vi "GEA2_ICP_Washer_SM.vi"(0 "ComPort":refnum<visa-resource-name>="COM1", 1 "Destination Address":u8=37 format="%.0x", 2 "Source Address":u8=229 format="%.0x", 3 "Mode":T2, 5 "Filter on Destination":bool, 7 "Read Bus Idle Timeout":u32=42, 9 "Byte Data":u8[](array[numeric]) format="%02x", 11 "Error In":errorcluster, 12 "Partial Message Start":u8[](array[numeric]) format="%02x", 13 "Command":u8(ring)=2 items=["CMD_Entry_Command", "CMD_Load_Control", "RQST_Input_Status", "CMD_LED_Control", "RQST_Encoder_Position_Status", "RQST_A2D_Status", "RQST_Switch_States_Status", "CMD_Buzzer_Control", "CMD_Shift_to_Spin", "CMD_Shift_to_Agitate", "RQST_Mode_Shift_Complete_Status", "CMD_Control_Inverter", "CMD_Spin_Action", "CMD_Agitate_Action", "RQST_Total_Switch_Status", "RQST_Total_Encoder_Status", "CMD_Test_Eeprom", "RQST_Eeprom_Test_Status", "CMD_Power_Mode", "RQST_Error_Status", "RQST_Get_Version", "CMD_Set_Personality", "RQST_Get_Personality", "CMD_Serial_Number", "RQST_Serial_Number_Status", "CMD_Model_Number", "RQST_Model_Number_Status", "CMD_Enter_Boot_Loader", "CMD_Enable_Debug_Log"]) -> (4 "Good Responses":cluster{"Bytes Data":u8[]}[](array[cluster]) {"Bytes Data" format="%02x"}, 10 "WriteOK":bool, 14 "Partial Message Out":u8[](array[numeric]) format="%.0x", 15 "Error Out":errorcluster)   [LabVIEW 2011]
uses:
  GEA2 Washer Interface Ctrl.ctl
  Dryer Wilt/Dryer Commands.ctl
  Hybrid Water Heater/HEWH Error Enumeration.ctl
  <vilib>/Instr/_visa.llb/VISA Configure Serial Port (Instr).vi
panel:
  in  "Read Continuous":bool
  out "CRC Match":bool
  in  "Tab Control":T1(tab)
  in  "Send Command":bool
  out "Command Bytes":u8[](array[numeric])=[226, 96, 8, 128, 86, 123, 137, 227] format="%.0x"
  out "Info":string
  in  "Read?":bool
  out "Length":u8
  out "Source Read":u8 format="%.0x"
  out "Destination Read":u8 format="%.0x"
  out "DataReturned":u8[](array[numeric]) format="%.0x"
  out "ReadArray":u8[](array[numeric]) format="%.0x"
  out "Bytes At Port":u32=40
  out "CRCRead":u8[](array[numeric]) format="%.0x"
  out "CRC Calc":u8[](array[numeric]) format="%.0x"
  out "Timeout":bool
  out "Num Messages":dbl
  out "Read Message Count":dbl
  out "CRCArray":u8[](array[numeric]) format="%.0x"
  out "Time Array":i32[](array[numeric])
  out "Tdiff":i32[](array[numeric])
  out "tStart":u32
  out "State Array":string[](array[string])
  out "Total mS":i32
  in  "Debug":bool
  out "Read_ACK":bool
  out "Message for Me":bool
  out "Partial Message":bool
  out "Current Start of Message Index":i32
  in  "Exit":bool
  # "Use only in Send Byte\nData Mode"
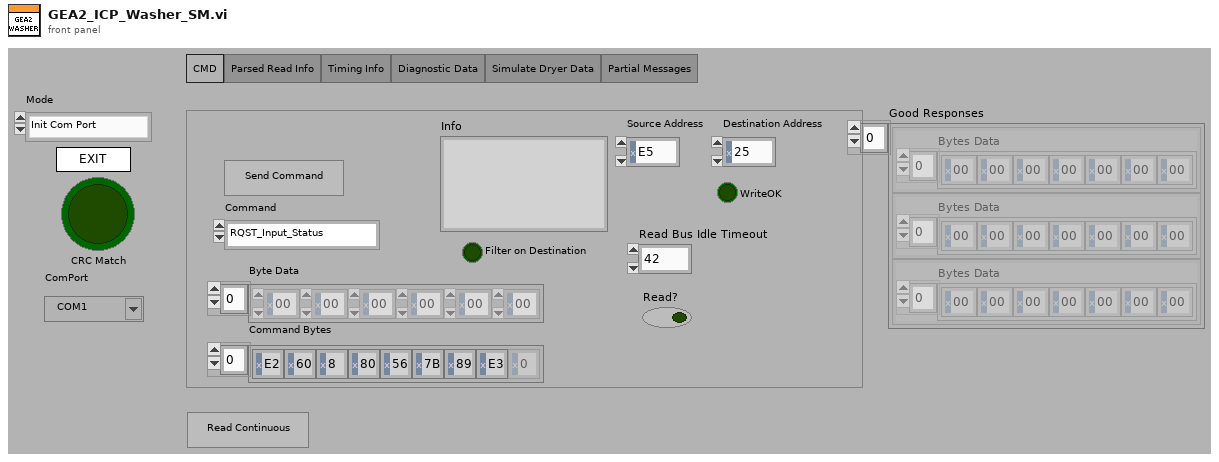
[diagram p1: front panel]
types:
  T1 = enum32{"CMD", "Parsed Read Info", "Timing Info", "Diagnostic Data", "Simulate Dryer Data", "Partial Messages"}
  T2 = typedef "GEA2 Washer Interface Ctrl.ctl" = enum16{"Init Com Port", "SendCMD", "ReadPort", "Close Port", "Send Byte Data", "Read Continuous"}
  T3 = enum32{"invalid app kind", "Development System", "Run Time System", "Student Edition", "Embedded LabVIEW", "Evaluation", "Custom"}
  T4 = enum32{"Invalid", "Standard", "Closed", "Hidden", "Minimized", "Maximized"}
  T5 = typedef "HEWH Error Enumeration.ctl" = enum16{"No Error", "GEA2 Send ACK Mismatch", "GEA2 STX", "GEA2 ETX", "GEA2 CRC Mismatch", "GEA2 ReadACK", "RTD In Range Error", "Fail Mean Tank Temp", "No Flow Config Data Found", "Failed Flow During Purge", "Temp During Purge", "Confirm IF Stop Fail", "Init Draw: TC_1 Out of Range", "Flow = 0 During Draw after 20s"}
  T6 = typedef "Dryer Commands.ctl" = u8
  T7 = cluster{"Core":cluster{"Current VI Reference":refnum<vi>, "Close Panel on Exit?":bool}, "ComPort":refnum<visa-resource-name>, "ReadArray":u8[], "Partial Message Start":u8[], "CRCArray":u8[], "Bytes Remaining":u8, "CRCRead":u8[], "CRC":bool, "Dryer Command":T6, "Error Out Flag":bool, "Bytes Data":u8[], "Current Read Index":i32, "Total Bytes Read":i32, "Reset MSG Count":bool, "ACK":bool, "ReadCM1Flag":bool, "ReadCM2Flag":bool, "Reset Pulse":bool, "Good Responses":cluster{"Bytes Data":u8[]}[]}
  T8 = cluster{"Current VI Reference":refnum<vi>, "Close Panel on Exit?":bool}
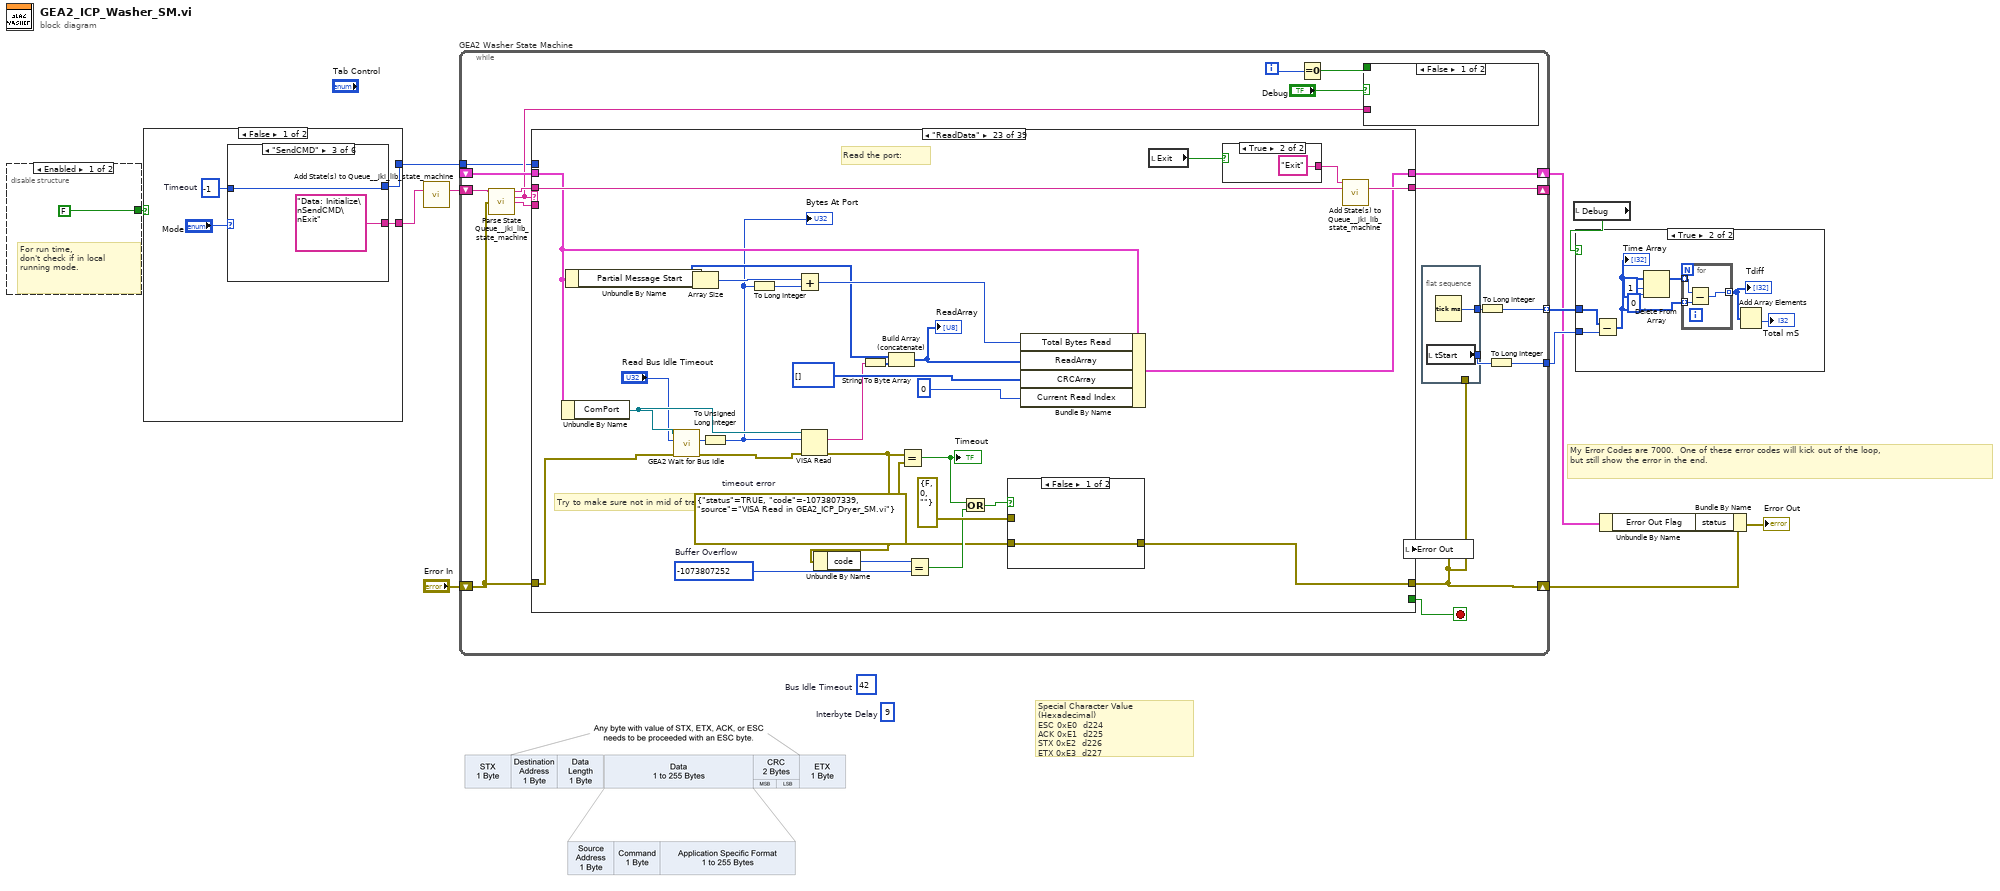
[diagram p0: block diagram]
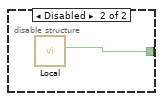
[diagram p2: hidden frame]
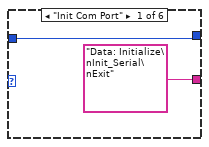
[diagram p3: hidden frame]
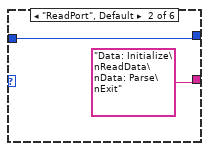
[diagram p4: hidden frame]
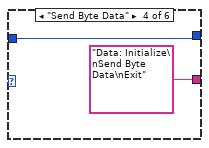
[diagram p5: hidden frame]
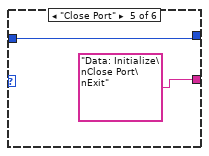
[diagram p6: hidden frame]
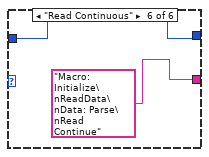
[diagram p7: hidden frame]
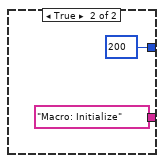
[diagram p8: hidden frame]
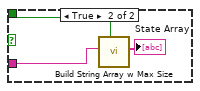
[diagram p10: hidden frame]
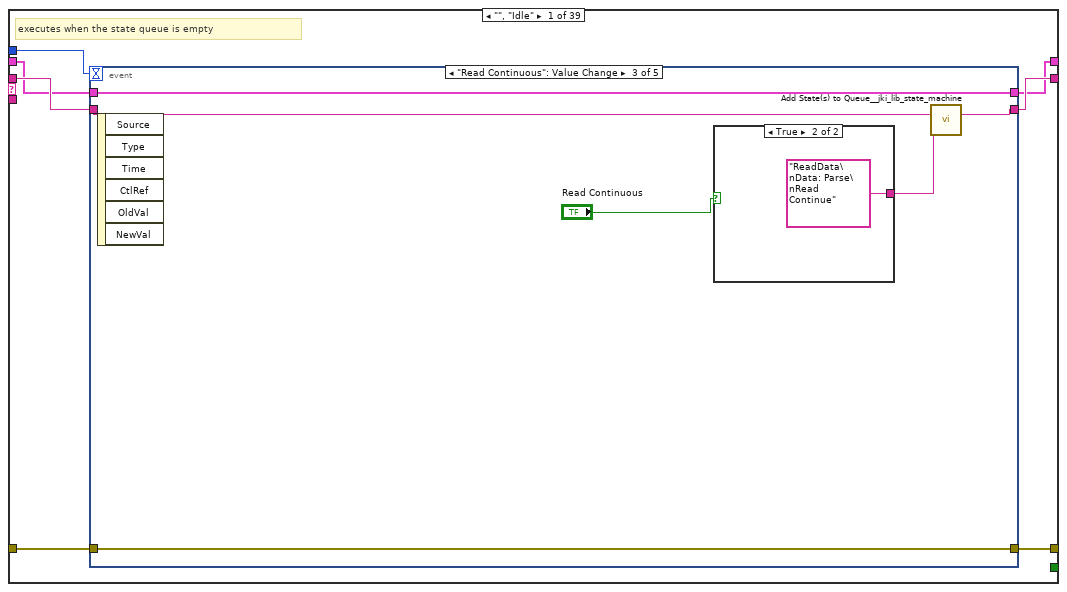
[diagram p11: hidden frame]
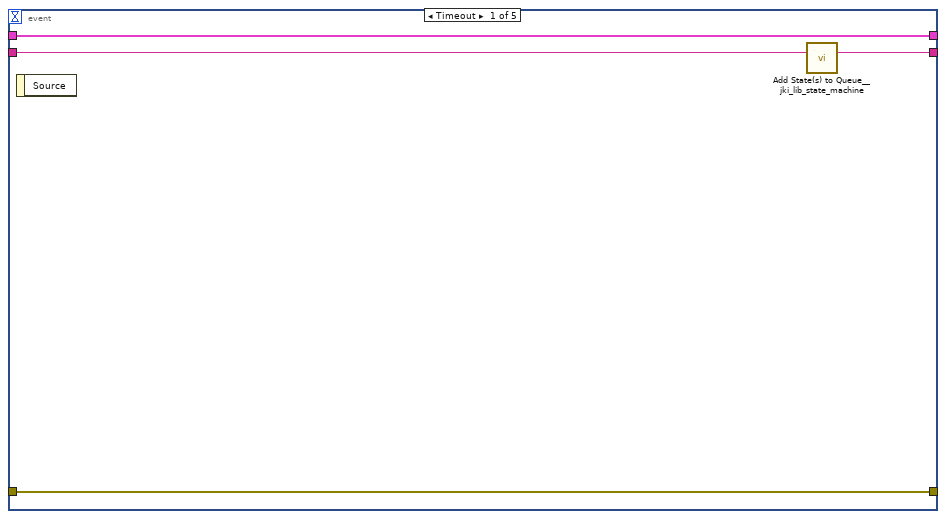
[diagram p12: hidden frame]
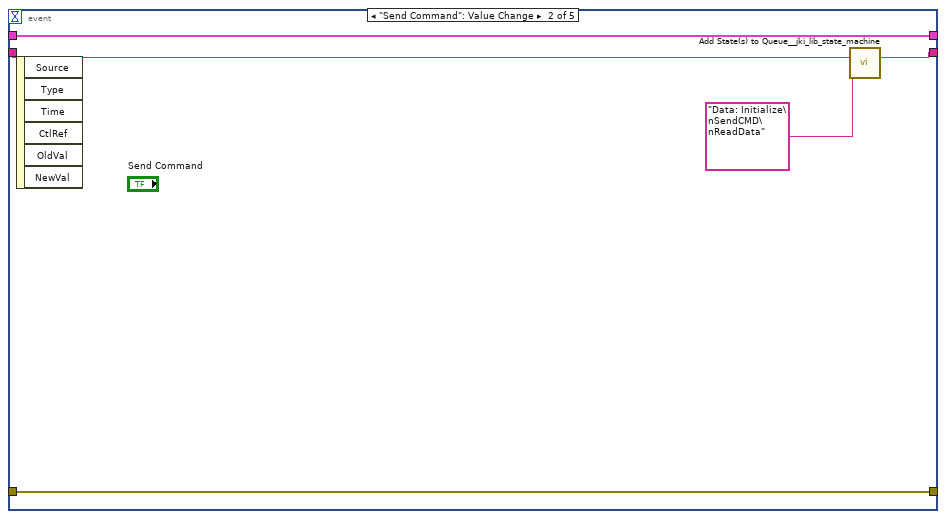
[diagram p13: hidden frame]
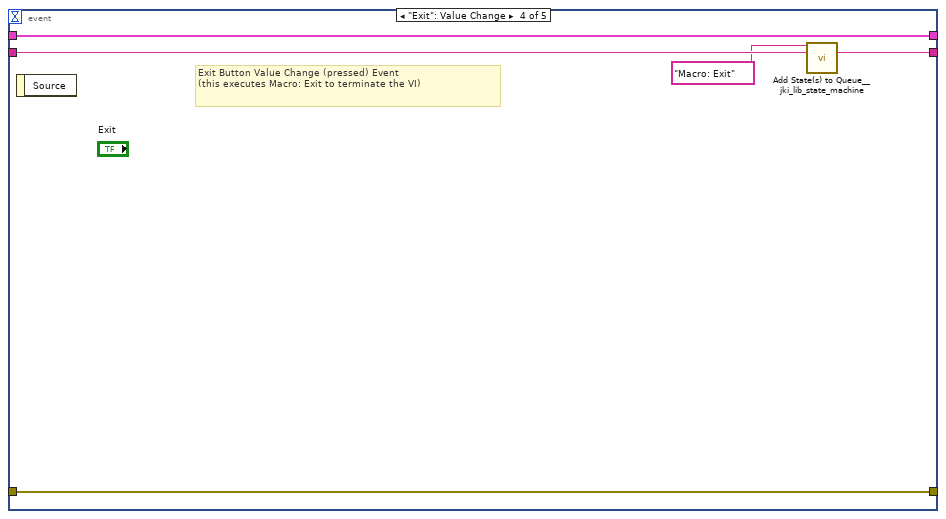
[diagram p15: hidden frame]
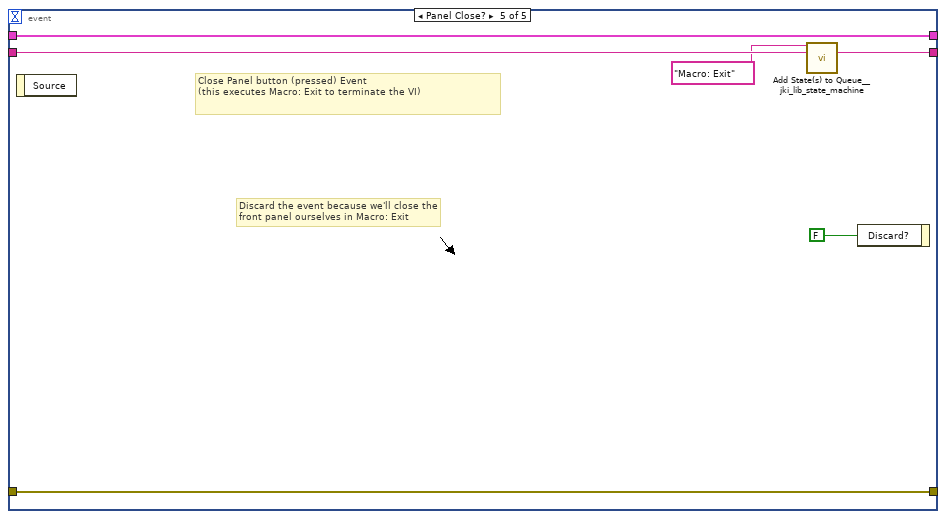
[diagram p16: hidden frame]
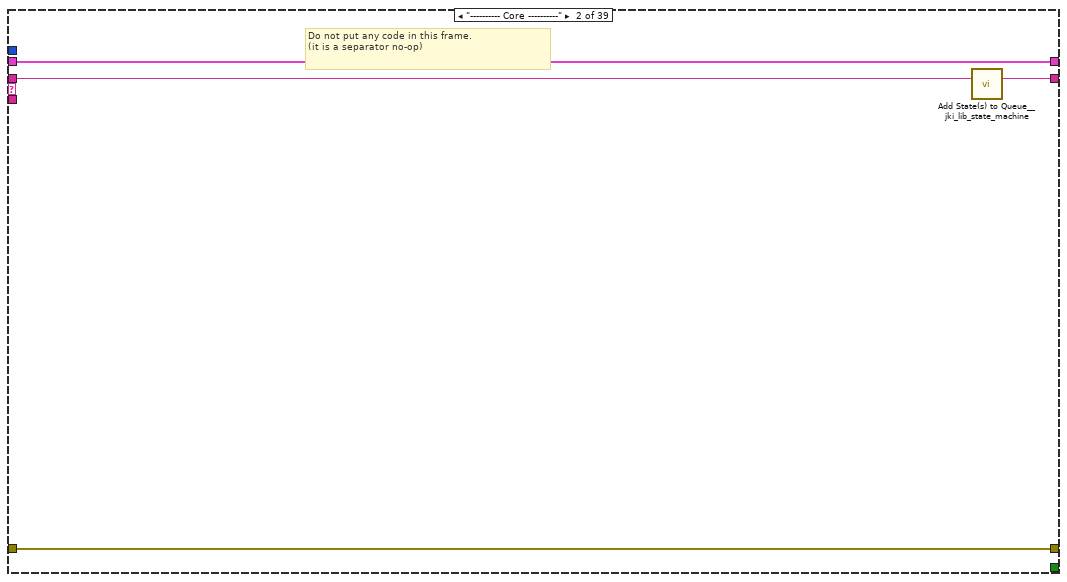
[diagram p17: hidden frame]
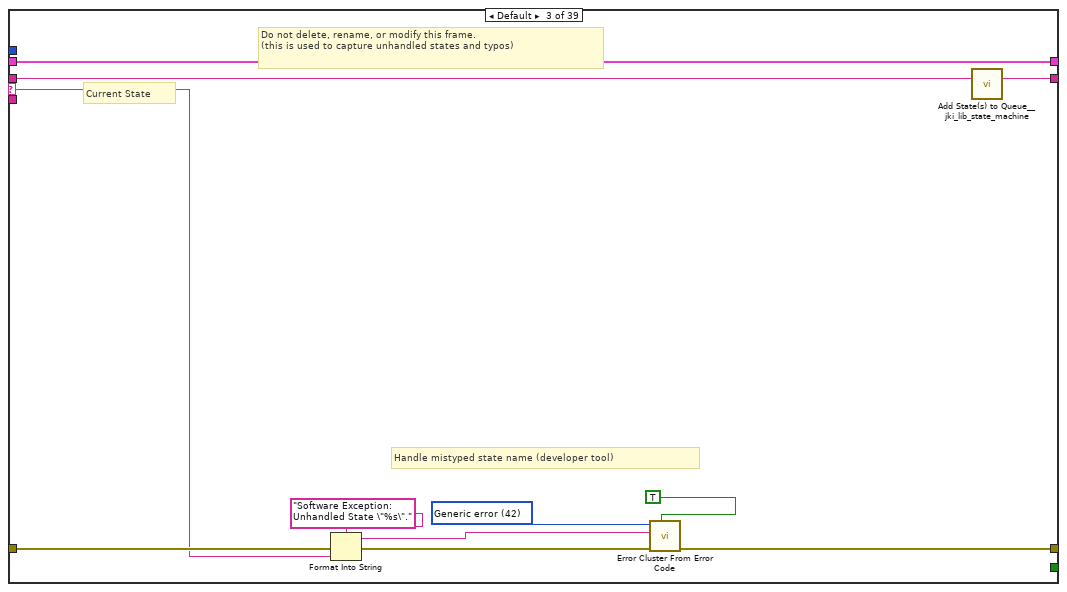
[diagram p18: hidden frame]
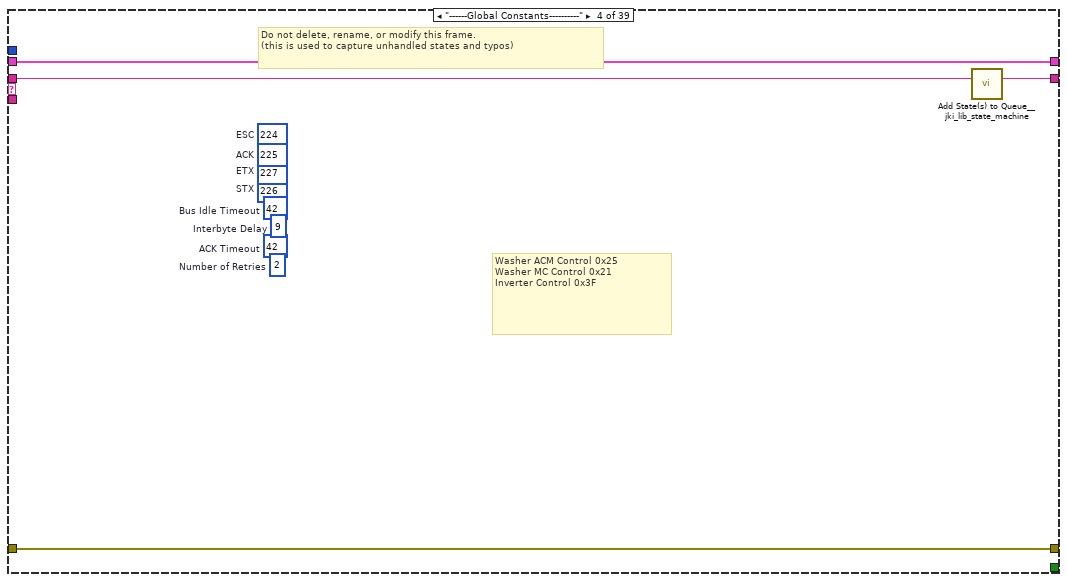
[diagram p19: hidden frame]
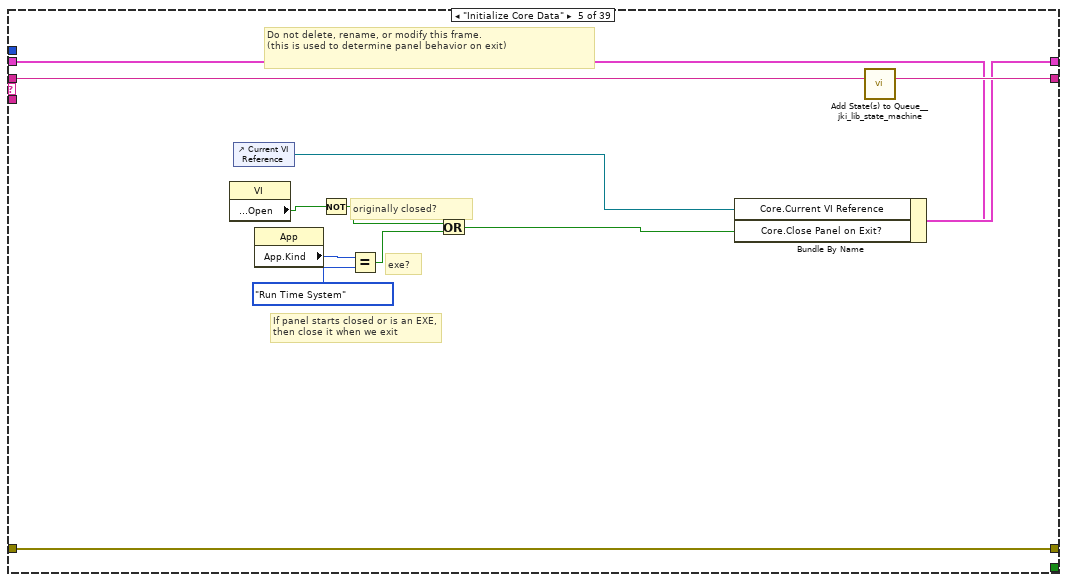
[diagram p20: hidden frame]
diagram:
  (unwired) 9  # Interbyte Delay
  (unwired) 42  # Bus Idle Timeout
  # "Special Character\tValue (Hexadecimal)\nESC\t0xE0  d224\nACK\t0xE1  d225\nSTX\t0xE2  d226\nETX\t0xE3  d227"
  # "My Error Codes are 7000.  One of these error codes will kick out of the loop,\nbut still show the error in the end."
  n1 = disable-structure shown="Enabled" {
    disable-tunnel: [FALSE w14] -> w1
    frame Enabled {
      # "For run time,\ndon't check if in local\nrunning mode."
    }
    frame Disabled {
      n2 = call "Local.vi"() -> ("Local?"=w14:bool)  [unwired: 11 in]
    }
  }
  n3 = case shown="False" w1 {
    tunnel: [w17 200 ("Timeout")] -> w4
    tunnel: [w15 "Macro: Initialize"] -> w2
    frame False {
      w16 = -1  # Timeout
      n4 = case shown="\"SendCMD\"" "Mode" {
        tunnel: ["Data: Initialize\nInit_Serial\nExit" "Data: Initialize\nReadData\nData: Parse\nExit" "Data: Initialize\nSendCMD\nExit" "Data: Initialize\nSend Byte Data\nExit" "Data: Initialize\nClose Port\nExit" "Macro: Initialize\nReadData\nData: Parse\nRead Continue"] -> w15
        tunnel: [w19 w21 w23 w25 w27 w30] -> w17
        tunnel: w16 -> [w19 w21 w23 w25 w27 w30]
        frame "Init Com Port" {
        }
        frame "ReadPort", Default {
        }
        frame "SendCMD" {
        }
        frame "Send Byte Data" {
        }
        frame "Close Port" {
        }
        frame "Read Continuous" {
        }
      }
    }
    frame True {
    }
  }
  n5 = call <vilib>:"Add State(s) to Queue__jki_lib_state_machine.vi"("State(s) in (\"\")"=w2) -> ("States Out"=w12:string)  [unwired: 14 in]
  n6 = while "GEA2 Washer State Machine" {
    shift-right: [w46] -> w6
    shift-left: _ -> [w45]
    shift-right: [w42] -> w10
    shift-left: "Error In" -> [w44]
    shift-right: [w43] -> _
    shift-left: w12 -> [w48]
    tunnel: [w39] -> w9 mode=indexing
    tunnel: [w38] -> w8
    tunnel: w4 -> [w36]
    i -> [w34]
    stop <- w47 stop-if-true
    n7 = call <vilib>:"Parse State Queue__jki_lib_state_machine.vi"("State Queue"=w48, "Error In (no error)"=w44) -> ("Remaining States"=w50:string, "Current State"=w37:string, "Arguments"=w49:string)  [unwired: 11 in]
    n8 = case shown="\"ReadData\"" w37 {
      selector: w37 -> [_ _ w94 _ _ _ _ _ _ _ _ _ _ _ _ _ _ _ _ _ _ _ _ _ _ _ _ _ _ _ _ _ _ _ _ _ _ _ _]
      tunnel: w50 -> [w62 w93 w98 w108 w120 w136 w138 w149 w178 w185 w190 w194 w200 w211 w237 w243 w248 w259 w276 w297 w346 w383 w415 w422 w431 w452 w484 w503 w547 w576 w597 w618 w634 w647 w660 w691 w713 w727 w734]
      tunnel: w49 -> [_ _ _ _ _ _ _ _ _ _ _ _ w195 w205 _ _ _ _ _ _ _ _ _ _ _ _ _ _ _ _ _ _ _ _ _ _ _ _ _]
      tunnel: w45 -> [w60 w90 w96 w106 w111 w132 w141 w146 _ w182 w187 w192 w198 w207 w234 w240 w245 w256 w273 w294 w323 w365 w397 w419 w425 w450 w482 w519 w545 w574 w595 w616 w629 w645 w655 w683 w702 w721 w732]
      tunnel: [w59 w91 w100 w105 w117 w134 w142 w147 w164 w180 w188 w191 w196 w208 w235 w241 w246 w257 w274 w295 w309 w355 w400 w420 w429 w447 w478 w516 w539 w570 w591 w612 w627 w642 w656 w689 w711 w725 w733] -> w42
      tunnel: w44 -> [w58 w91 w99 w105 w117 w128 w142 w147 w164 w183 w188 w191 w197 w209 w235 w241 w246 w257 w263 w290 w327 w369 w391 w420 w429 w445 w478 w516 w539 w570 w591 w612 w632 w639 w658 w689 w711 w725 w733]
      tunnel: [w61 w92 w97 w107 w119 w135 w143 w148 w177 w184 w189 w193 w199 w210 w236 w242 w247 w258 w275 w296 w345 w382 w414 w421 w430 w451 w483 w520 w546 w575 w596 w617 w633 w646 w659 w690 w712 w726 w735] -> w43
      tunnel: [_ _ _ _ _ _ w139 _ _ _ _ _ _ _ _ _ _ _ _ _ _ _ _ _ _ _ _ _ _ _ _ _ _ _ _ _ _ _ _] -> w47
      tunnel: [w57 w90 w96 w106 w118 w131 w141 w146 w176 w182 w187 w192 w198 w207 w234 w240 w245 w256 w272 w293 w323 w365 w407 w419 w424 w449 w481 w518 w544 w573 w594 w615 w628 w644 w655 w682 w701 w724 w732] -> w46
      tunnel: w36 -> [w56 _ _ _ _ _ _ _ _ _ _ _ _ _ _ _ _ _ _ _ _ _ _ _ _ _ _ _ _ _ _ _ _ _ _ _ _ _ _]
      frame "", "Idle" {
        # "executes when the state queue is empty"
        n9 = event shown="[2] \"Read Continuous\": Value Change" {
          selector: _ -> [_ _ _ _ _]
          dyn-events: _ -> [_ _ _ _ _]
          timeout: w56 -> [_ _ _ _ _]
          tunnel: w62 -> [w66 w69 w75 w83 w89]
          tunnel: [w65 w70 w76 w82 w88] -> w61
          tunnel: w60 -> [w63 w71 w77 w80 w86]
          tunnel: [w64 w67 w73 w81 w87] -> w59
          tunnel: w58 -> [w64 w67 w73 w81 w87]
          tunnel: [w63 w71 w77 w80 w86] -> w57
          event Timeout {
            n10 = event-data() -> ()  [unwired: 1 in, 1 out]
            n11 = call <vilib>:"Add State(s) to Queue__jki_lib_state_machine.vi"("State(s) in (\"\")"=w66) -> ("States Out"=w65:string)  [unwired: 14 in]
          }
          event "Send Command": Value Change {
            n12 = event-data() -> ()  [unwired: 1 in, 6 out]
            n13 = call <vilib>:"Add State(s) to Queue__jki_lib_state_machine.vi"("State(s) in (\"\")"=w69, "State(s) at Back (\"\")"="Data: Initialize\nSendCMD\nReadData") -> ("States Out"=w70:string)  [unwired: 13 in]
          }
          event "Read Continuous": Value Change {
            n14 = event-data() -> ()  [unwired: 1 in, 6 out]
            n15 = case shown="True" "Read Continuous" {
              tunnel: [_ "ReadData\nData: Parse\nRead Continue"] -> w74
              frame False {
              }
              frame True {
              }
            }
            n16 = call <vilib>:"Add State(s) to Queue__jki_lib_state_machine.vi"("State(s) in (\"\")"=w75, "State(s) at Back (\"\")"=w74) -> ("States Out"=w76:string)  [unwired: 13 in]
          }
          event "Exit": Value Change {
            # "Exit Button Value Change (pressed) Event\n(this executes Macro: Exit to terminate the VI)"
            n17 = event-data() -> ()  [unwired: 1 in, 1 out]
            n18 = call <vilib>:"Add State(s) to Queue__jki_lib_state_machine.vi"("State(s) in Front (\"\")"="Macro: Exit", "State(s) in (\"\")"=w83) -> ("States Out"=w82:string)  [unwired: 13 in]
          }
          event Panel Close? {
            # "Discard the event because we'll close the front panel ourselves in Macro: Exit"
            # "Close Panel button (pressed) Event\n(this executes Macro: Exit to terminate the VI)"
            n19 = event-data() -> ()  [unwired: 1 in, 1 out]
            n20 = call <vilib>:"Add State(s) to Queue__jki_lib_state_machine.vi"("State(s) in Front (\"\")"="Macro: Exit", "State(s) in (\"\")"=w89) -> ("States Out"=w88:string)  [unwired: 13 in]
            n21 = event-data("Discard?"=FALSE) -> ()  [unwired: 1 in, 1 out]
          }
        }
      }
      frame "---------- Core ----------" {
        # "Do not put any code in this frame.\n(it is a separator no-op)"
        n22 = call <vilib>:"Add State(s) to Queue__jki_lib_state_machine.vi"("State(s) in (\"\")"=w93) -> ("States Out"=w92:string)  [unwired: 14 in]
      }
      frame Default {
        w103 = 42 items=["No error", "Argument error", "Memory is full", "Out of zone", "End of file", "File already open", "Generic file I/O error", "File not found", "File permission error", "Disk is full", "Duplicate path", "Too many files open", "System feature not enabled", "Resource file not found", "Cannot add resource", "Resource not found", "Image not found", "Image memory error", "Pen does not exist", "Config type invalid", "Config token not found", "Config parse error", "Config memory error", "Bad external code format", "Bad external code offset", "External code not present", "Null window", "Destroy window error", "Null menu", "Print aborted", "Bad print record", "Print driver error", "Windows error during printing", "Memory error during printing", "Print dialog error", "Generic print error", "Invalid device refnum", "Device not found", "Device parameter error", "Device unit error", "Cannot open device", "Device call aborted", "Generic error", "Cancelled by user", "Object ID too low", "Object ID too high", "Object not in heap", "Unknown heap", "Unknown object (invalid DefProc)", "Unknown object (DefProc not in table)", "Message out of range", "Invalid (null) method", "Unknown message", "Manager call not supported", "Bad address", "Network operation in progress", "Network operation timed out", "Connection is busy", "Network attribute not supported", "Network error", "Address in use", "System out of memory", "Connection aborted", "Connection refused", "Not connected", "Already connected", "Connection closed", "Initialization error (interapplication manager)", "Bad occurrence", "Wait on unbound occurrence handler", "Occurrence queue overflow", "Datalog type conflict", "Unused", "Unrecognized type (interapplication manager)", "Memory corrupt", "Failed to make temporary DLL", "Old CIN version", "Drag socket not found", "Failed to load drop-object", "Failed to register OLE object", "Failed to release OLE object", "Format specifier type mismatch", "Unknown format specifier", "Too few format specifiers", "Too many format specifiers", "Scan failed", "Newer CIN version", "Error converting to variant", "Runtime menu error", "Password tampered", "Variant attribute not found", "Incompatible variant data type", "Event data is not available", "Event Store is not present", "Occurrence is not found", "Event Queue is not created", "Event info is not available", "Refnum passed is NULL", "Error retrieving Class GUID", "Error retrieving CoClass GUID", "Error retrieving TypeLib GUID.", "Bad built application magic bytes.", "Specific driver is different from the specific driver associated with the Logical Name.", "There is no session opened to the class driver.", "Max Error", "MAX - Error with config objects", "MAX - Error loading configuration", "MAX - Group not supported"]
        # "Current State"
        # "Do not delete, rename, or modify this frame.\n(this is used to capture unhandled states and typos)"
        # "Handle mistyped state name (developer tool)"
        n23 = Format Into String(format string="Software Exception: Unhandled State \"%s\"." ("message"), error in=w99, w94) -> (resulting string=w102:string, error out=w101:errorcluster)  [unwired: 1 in]
        n24 = call <vilib>:"Error Cluster From Error Code.vi"("show call chain? (False)"=TRUE, "error in (no error)"=w101, "error message (\"\")"=w102, "error code (0)"=w103) -> ("error out"=w100:errorcluster)  [unwired: 5 in]
        n25 = call <vilib>:"Add State(s) to Queue__jki_lib_state_machine.vi"("State(s) in (\"\")"=w98) -> ("States Out"=w97:string)  [unwired: 14 in]
      }
      frame "------Global Constants----------" {
        (unwired) u8 224  # ESC
        (unwired) 2  # Number of Retries
        (unwired) 42  # ACK Timeout
        (unwired) 9  # Interbyte Delay
        (unwired) 42  # Bus Idle Timeout
        (unwired) u8 226  # STX
        (unwired) u8 227  # ETX
        (unwired) u8 225  # ACK
        # "Washer ACM Control\t0x25\nWasher MC Control\t0x21\nInverter Control\t0x3F"
        # "Do not delete, rename, or modify this frame.\n(this is used to capture unhandled states and typos)"
        n26 = call <vilib>:"Add State(s) to Queue__jki_lib_state_machine.vi"("State(s) in (\"\")"=w108) -> ("States Out"=w107:string)  [unwired: 14 in]
      }
      frame "Initialize Core Data" {
        # "Do not delete, rename, or modify this frame.\n(this is used to determine panel behavior on exit)"
        # "originally closed?"
        # "exe?"
        # "If panel starts closed or is an EXE, then close it when we exit"
        n27 = property class="VI"() -> ("Front Panel.Open"=w116:bool)  [unwired: 2 in, 2 out]
        n28 = control-ref of="Current VI Reference"() -> (w109:refnum<vi>)
        n29 = property class="App"() -> ("App.Kind"=w115:T3)  [unwired: 2 in, 2 out]
        n30 = Not(x=w116) -> (.not. x?=w113:bool)
        n31 = Equal?(x=w115, y=T3."Run Time System" ("Application:Kind")) -> (x = y?=w112:bool)
        n32 = Or(x=w113, y=w112) -> (x .or. y?=w110:bool)
        n33 = Bundle By Name(cluster=w111, "Core.Current VI Reference"=w109, "Core.Close Panel on Exit?"=w110) -> (w118:T7)
        n34 = call <vilib>:"Add State(s) to Queue__jki_lib_state_machine.vi"("State(s) in (\"\")"=w120) -> ("States Out"=w119:string)  [unwired: 14 in]
      }
      frame "Error Handler" {
        # "State Machine Does not handle having an error status = true."
        n35 = local read "ReadArray"() -> (w125:u8[])
        n36 = Unbundle By Name(w128) -> ("source"=w127:string)
        n37 = Number To Hexadecimal String(2:w125) -> (0:w124:string[])  [unwired: 1 in]
        n38 = Array To Spreadsheet String(array=w124, 3:"" ("format string")) -> (spreadsheet string=w122:string)  [unwired: 1 in]
        n39 = Concatenate Strings(w127, ":: BYTES :: " ("string"), w122) -> (w121:string)
        n40 = Bundle By Name(cluster=w132, "Error Out Flag"=TRUE) -> (w131:T7)
        n41 = Bundle By Name(cluster=w128, "source"=w121, "status"=FALSE) -> (w134:errorcluster)
        n42 = call <vilib>:"Add State(s) to Queue__jki_lib_state_machine.vi"("State(s) in Front (\"\")"="Exit", "State(s) in (\"\")"=w136) -> ("States Out"=w135:string)  [unwired: 13 in]
      }
      frame "Exit" {
        # "Do not put any code in this frame.\n(No errors that occur here will be handled.)"
        n43 = local read "Mode"() -> (w140:T2)
        n44 = case shown="\"Init Com Port\", Default" w140 {
          tunnel: [TRUE] -> w139
          tunnel: w138 -> [w144]
          tunnel: [w144] -> w137
          frame "Init Com Port", Default {
          }
        }
        n45 = call <vilib>:"Add State(s) to Queue__jki_lib_state_machine.vi"("State(s) in (\"\")"=w137) -> ("States Out"=w143:string)  [unwired: 14 in]
      }
      frame "---------- Data ----------" {
        # "Do not put any code in this frame.\n(It is a separator no-op. You can make a copy of this frame to create a new Data frame)"
        n46 = call <vilib>:"Add State(s) to Queue__jki_lib_state_machine.vi"("State(s) in (\"\")"=w149) -> ("States Out"=w148:string)  [unwired: 14 in]
      }
      frame "Data: Initialize" {
        w150 = cluster{"Bytes Data":u8[]}[] []  # Good Responses
        w151 = FALSE ("Start Pressed")
        w154 = TRUE  # Reset Pulse
        w156 = FALSE  # ReadCM2Flag
        w157 = FALSE  # ReadCM1Flag
        w158 = FALSE  # ACK
        w159 = TRUE  # Reset MSG Count
        w160 = 0  # Total Bytes Read
        w161 = 0  # Current Read Index
        w165 = u8 0 ("Length")
        w166 = T6 3 items=["Eval_Mode_Entry_CC1", "Eval_Mode_Entry_CC2", "Eval_Mode_Continue", "Get_Diagnostic_Info"]  # Dryer Command
        w167 = u8[] []  # Bytes Data
        w168 = T8 {"Current VI Reference"=refnum, "Close Panel on Exit?"=FALSE}  # Core
        w155 = FALSE ("CRC Match")
        w169 = FALSE  # Error Out Flag
        w170 = FALSE  # CRC
        w171 = u8[] []  # CRCRead
        w172 = u8 0  # Bytes Remaining
        w173 = u8[] []  # CRCArray
        w174 = u8[] []  # ReadArray
        # "Don' Run with Err In"
        # "Initialize the shift-register data, here.\n(data names are defined by what you wire into the bundle function)"
        n47 = local write "Num Messages"(0.0 ("Num Messages")) -> ()
        n48 = local write "Read Continuous"(w151) -> ()
        n49 = local write "Exit"(w151) -> ()
        n50 = local write "Bytes At Port"(u32 0 ("Bytes At Port")) -> ()
        n51 = local write "Source Read"(w165) -> ()
        n52 = local write "Length"(w165) -> ()
        n53 = local write "Message for Me"(w155) -> ()
        n54 = local write "Partial Message"(w155) -> ()
        n55 = local write "CRC Match"(w155) -> ()
        n56 = local write "Read_ACK"(w155) -> ()
        n57 = local write "WriteOK"(w155) -> ()
        n58 = local write "Timeout"(w155) -> ()
        n59 = Bundle("Core"=w168, "ComPort"="ComPort", "ReadArray"=w174, "Partial Message Start"="Partial Message Start", "CRCArray"=w173, "Bytes Remaining"=w172, "CRCRead"=w171, "CRC"=w170, "Dryer Command"=w166, "Error Out Flag"=w169, "Bytes Data"=w167, "Current Read Index"=w161, "Total Bytes Read"=w160, "Reset MSG Count"=w159, "ACK"=w158, "ReadCM1Flag"=w157, "ReadCM2Flag"=w156, "Reset Pulse"=w154, "Good Responses"=w150) -> (w176:T7)  [unwired: 1 in]
        n60 = case shown="No Error" w164 {
          tunnel: [_ "Exit"] -> w163
          frame No Error {
          }
          frame Error {
          }
        }
        n61 = call <vilib>:"Add State(s) to Queue__jki_lib_state_machine.vi"("State(s) in Front (\"\")"=w163, "State(s) in (\"\")"=w178) -> ("States Out"=w177:string)  [unwired: 13 in]
      }
      frame "Data: Cleanup" {
        # "Cleanup any data and references, here.\n(this is called automatically, by the Macro: Exit)"
        n62 = Unbundle By Name(w182) -> ("Core.Current VI Reference"=w181:refnum<vi>)
        n63 = Close Reference(reference=w181, error in (no error)=w183) -> (error out=w180:errorcluster)
        n64 = case shown="Error" w180 {
          frame No Error {
          }
          frame Error {
            n65 = String Length(string="") -> ()  [unwired: 1 out]
          }
        }
        n66 = call <vilib>:"Add State(s) to Queue__jki_lib_state_machine.vi"("State(s) in (\"\")"=w185) -> ("States Out"=w184:string)  [unwired: 14 in]
      }
      frame "---------- UI ----------" {
        # "Do not put any code in this frame.\n(It is a separator no-op. You can make a copy of this frame to create a new UI frame)"
        n67 = call <vilib>:"Add State(s) to Queue__jki_lib_state_machine.vi"("State(s) in (\"\")"=w190) -> ("States Out"=w189:string)  [unwired: 14 in]
      }
      frame "UI: Initialize" {
        # "Initialize the User Interface, here.\n(this is called automatically, by the Macro: Init)"
        n68 = call <vilib>:"Add State(s) to Queue__jki_lib_state_machine.vi"("State(s) in (\"\")"=w194) -> ("States Out"=w193:string)  [unwired: 14 in]
      }
      frame "UI: Cursor Set" {
        # "Argument"
        # "Set and Unset Cursor Busy.\n(Usage: \"UI: Cursor Set >> Busy|Idle\")"
        n69 = case shown="\"Idle\", Default" w195 {
          tunnel: w197 -> [w202 w204]
          tunnel: [w201 w203] -> w196
          frame "Idle", Default {
            n70 = call <vilib>:"Unset Busy.vi"("error in (no error)"=w202) -> ("error out"=w201:errorcluster)  [unwired: 10 in]
          }
          frame "Busy" {
            n71 = call <vilib>:"Set Busy.vi"("error in (no error)"=w204) -> ("error out"=w203:errorcluster)  [unwired: 9 in, 1 out]
          }
        }
        n72 = call <vilib>:"Add State(s) to Queue__jki_lib_state_machine.vi"("State(s) in (\"\")"=w200) -> ("States Out"=w199:string)  [unwired: 14 in]
      }
      frame "UI: Front Panel State" {
        # "Argument"
        # "Set Front Panel Open or Closed\n(Usage: \"UI: Front Panel State >> Open|Close\")"
        n73 = Unbundle By Name(w207) -> ("Core.Current VI Reference"=w206:refnum<vi>)
        n74 = case shown="\"Close\"" w205 {
          tunnel: w209 -> [w215 w228]
          tunnel: [w217 w229] -> w208
          tunnel: w206 -> [w216 w226]
          frame "Open", Default {
            n75 = property class="VI"(reference=w216, error in=w215) -> (reference out=w213:refnum<vi>, error out=w214:errorcluster, "Front Panel.Open"=w212:bool)
            n76 = case shown="False" w212 {
              tunnel: [w220 w223] -> w217
              tunnel: w214 -> [w219 w223]
              tunnel: w213 -> [w218 _]
              frame False {
                n77 = invoke class="VI" method="FP.Open"(reference=w218, error in=w219, "Activate"=TRUE, "State"=T4."Standard") -> (error out=w220:errorcluster)  [unwired: 1 in, 4 out]
              }
              frame True {
              }
            }
          }
          frame "Close" {
            n78 = property class="VI"(reference=w226, error in=w228) -> (reference out=w225:refnum<vi>, error out=w227:errorcluster, "Front Panel.Open"=w224:bool)
            n79 = case shown="True" w224 {
              tunnel: [w230 w233] -> w229
              tunnel: w227 -> [w230 w232]
              tunnel: w225 -> [_ w231]
              frame False {
              }
              frame True {
                n80 = invoke class="VI" method="FP.Close"(reference=w231, error in=w232) -> (error out=w233:errorcluster)  [unwired: 1 in, 2 out]
              }
            }
          }
        }
        n81 = call <vilib>:"Add State(s) to Queue__jki_lib_state_machine.vi"("State(s) in (\"\")"=w211) -> ("States Out"=w210:string)  [unwired: 14 in]
      }
      frame "---------- Macro ----------" {
        # "Do not put any code in this frame.\n(It is a separator no-op. You can make a copy of this frame to create a new Macro frame)"
        n82 = call <vilib>:"Add State(s) to Queue__jki_lib_state_machine.vi"("State(s) in (\"\")"=w237) -> ("States Out"=w236:string)  [unwired: 14 in]
      }
      frame "Macro: Initialize" {
        w239 = "Data: Initialize\nInitialize Core Data\nUI: Initialize\nUI: Front Panel State >> Open\nInit_Serial"  # Data: Initialize Initialize Core Data UI: Initialize UI: Front Panel State >> Open Init_Serial
        # "Initialization Macro\n(This is called once, when the VI starts)"
        n83 = Tick Count (ms)() -> (millisecond timer value=→"tStart":u32)
        n84 = call <vilib>:"Add State(s) to Queue__jki_lib_state_machine.vi"("State(s) in Front (\"\")"=w239, "State(s) in (\"\")"=w243) -> ("States Out"=w242:string)  [unwired: 13 in]
      }
      frame "Macro: Exit" {
        # "Exit Macro\n(This is called once, when the VI exits)"
        n85 = disable-structure shown="Enabled" {
          disable-tunnel: w245 -> [w255 _]
          disable-tunnel: [w250 _] -> w244
          frame Enabled {
            n86 = Unbundle By Name(w255) -> ("Core.Close Panel on Exit?"=w249:bool)
            n87 = Select(t="UI: Front Panel State >> Close", s=w249, f="") -> (s? t:f=w252:string)
            n88 = call <vilib>:"Add State(s) to Queue__jki_lib_state_machine.vi"("State(s) in (\"\")"=w252, "State(s) at Back (\"\")"="Data: Cleanup\nExit") -> ("States Out"=w250:string)  [unwired: 13 in]
          }
          frame Disabled {
          }
        }
        n89 = call <vilib>:"Add State(s) to Queue__jki_lib_state_machine.vi"("State(s) in Front (\"\")"=w244, "State(s) in (\"\")"=w248) -> ("States Out"=w247:string)  [unwired: 13 in]
      }
      frame "---------- New Category ----------" {
        # "Template Separator\n(You can make a copy of, or modify, this frame)"
        n90 = call <vilib>:"Add State(s) to Queue__jki_lib_state_machine.vi"("State(s) in (\"\")"=w259) -> ("States Out"=w258:string)  [unwired: 14 in]
      }
      frame "Init_Serial" {
        (unwired) u32 8  # ACK Timeout
        w268 = u16 0 items=["None", "XON/XOFF", "RTS/CTS", "XON/XOFF & RTS/CTS", "DTR/DSR", "XON/XOFF & DTR/DSR"] ("flow control (0:none)")
        w267 = u16 10 items=["1.0"=10, "1.5"=15, "2.0"=20] ("stop bits (10: 1 bit)")
        # "Note that long reads weren't completeing in 8 ms."
        # "skip error handle routine"
        # "Assumes that if the serial port is 19200, then it is all ok."
        # "Your code here.\n(You can make a copy of, or modify, this frame)"
        n91 = Unbundle By Name(w273) -> ("ComPort"=w262:refnum<visa-resource-name>)
        n92 = call-poly "VISA Configure Serial Port"("VISA resource name"=w262, "timeout (10sec)"=u32 20, "Enable Termination\nChar (T)"=FALSE ("Enable Termination\nChar (T)"), "baud rate (9600)"=u32 19200, "data bits (8)"=u16 8, "parity (0:none)"=enum16{"None", "Odd", "Even", "Mark", "Space"}."None", "error in (no error)"=w263, "stop bits (10: 1 bit)"=w267, "flow control (0:none)"=w268) -> ("VISA resource name out"=w270:refnum<visa-resource-name>, "error out"=w261:errorcluster)  [unwired: 5 in]
        n93 = case shown="Error" w261 {
          selector: w261 -> [w277 w284]
          tunnel: w273 -> [w281 w288]
          tunnel: [w280 w287] -> w272
          tunnel: w270 -> [w279 _]
          tunnel: ["" ("State(s) in Front (\"\")") "Exit" ("State(s) in Front (\"\")")] -> w271
          tunnel: [w277 w282] -> w274
          frame No Error {
            n94 = Bundle By Name(cluster=w281, "ComPort"=w279) -> (w280:T7)
          }
          frame Error {
            n95 = Bundle By Name(cluster=w288, "Error Out Flag"=TRUE) -> (w287:T7)
            n96 = Bundle By Name(cluster=w284, "status"=FALSE) -> (w282:errorcluster)
          }
        }
        n97 = call <vilib>:"Add State(s) to Queue__jki_lib_state_machine.vi"("State(s) in Front (\"\")"=w271, "State(s) in (\"\")"=w276) -> ("States Out"=w275:string)  [unwired: 13 in]
      }
      frame "Close Port" {
        # "skip error handle routine"
        # "Assumes that if the serial port is 19200, then it is all ok."
        # "Your code here.\n(You can make a copy of, or modify, this frame)"
        n98 = Unbundle By Name(w294) -> ("ComPort"=w289:refnum<visa-resource-name>)
        n99 = VISA Close(VISA resource name=w289, error in (no error)=w290) -> (error out=w291:errorcluster)
        n100 = case shown="Error" w291 {
          selector: w291 -> [w299 w303]
          tunnel: w294 -> [w298 w307]
          tunnel: [w298 w306] -> w293
          tunnel: ["" ("State(s) in Front (\"\")") "Macro: Exit" ("State(s) in Front (\"\")")] -> w292
          tunnel: [w299 w301] -> w295
          frame No Error {
          }
          frame Error {
            n101 = Bundle By Name(cluster=w307, "Error Out Flag"=TRUE) -> (w306:T7)
            n102 = Bundle By Name(cluster=w303, "status"=FALSE) -> (w301:errorcluster)
          }
        }
        n103 = call <vilib>:"Add State(s) to Queue__jki_lib_state_machine.vi"("State(s) in Front (\"\")"=w292, "State(s) in (\"\")"=w297) -> ("States Out"=w296:string)  [unwired: 13 in]
      }
      frame "SendCMD" {
        w315 = u32 8  # Bus Idle Timeout
        w325 = u8 225  # ACK
        w333 = u8 227  # ETX
        w336 = u8 226  # STX
        # "Washer ACM Control\t0x25\nWasher MC Control\t0x21\nInverter Control\t0x3F"
        n104 = Unbundle By Name(w323) -> ("ComPort"=w312:refnum<visa-resource-name>)
        n105 = call "Washer_DSM_CMD.vi"("Command"="Command") -> ("Info"=→"Info":string, "CMD Byte"=w337:u8[])  [unwired: 9 in]
        n106 = Array Size(array=w337) -> (size(s)=w343:i32)
        n107 = Array Size(array="Byte Data") -> (size(s)=w341:i32)
        n108 = Compound Arithmetic op=ADD(7 ("x"), w343, w341) -> (w339:i32)
        n109 = To Unsigned Byte Integer(number=w339) -> (unsigned 8bit integer=w340:u8)
        n110 = Build Array (concatenate)("Destination Address", w340, "Source Address", w337, "Byte Data") -> (w335:u8[])
        n111 = call "crc16-ccitt (x1021).vi"("unsigned byte array"=w335) -> ("CRC"=w334:u8[])  [unwired: 9 in, 1 out]
        n112 = call "HEWH Command Needs Read.vi"("Command"="Command") -> ("RQST"=w322:bool)  [unwired: 13 in, 1 out]
        n113 = Build Array (concatenate)(w336, w335, w334, w333) -> (w319:u8[])
        n114 = call "GEA2 Add ESC Char.vi"("Message"=w319) -> ("Message Out"=w318:u8[])  [unwired: 14 in]
        "Command Bytes" <- w318
        n115 = call "GEA2 Wait for Bus Idle.vi"("Error In"=w327, "Idle Time"=w315, "ComPort"=w312) -> ("error out"=w314:errorcluster)  [unwired: 7 in, 1 out]
        n116 = Byte Array To String(unsigned byte array=w318) -> (string=w320:string)
        n117 = Array Size(array=w318) -> (size(s)=w329:i32)
        n118 = VISA Flush I/O Buffer(VISA resource name=w312, error in (no error)=w314) -> (error out=w313:errorcluster)  [unwired: 1 in, 1 out]
        n119 = Increment(x=w329) -> (x+1=w326:i32)
        n120 = VISA Write(VISA resource name=w312, write buffer=w320, error in (no error)=w313) -> (VISA resource name out=w332:refnum<visa-resource-name>, error out=w331:errorcluster)  [unwired: 1 out]
        n121 = To Unsigned Long Integer(number=w326) -> (unsigned 32bit integer=w317:u32)
        n122 = Build Array (concatenate)(w318, w325) -> (w324:u8[])
        n123 = Byte Array To String(unsigned byte array=w324) -> (string=w328:string)
        n124 = VISA Read(VISA resource name=w332, byte count=w317, error in (no error)=w331) -> (read buffer=w311:string, error out=w309:errorcluster)  [unwired: 2 out]
        n125 = case shown="True" w322 {
          tunnel: ["" "ReadData\nData: Parse\n"] -> w321
          frame False {
          }
          frame True {
          }
        }
        n126 = Equal?(x=w328, y=w311) -> (x = y?=→"WriteOK":bool)
        n127 = call <vilib>:"Add State(s) to Queue__jki_lib_state_machine.vi"("State(s) in Front (\"\")"=w321, "State(s) in (\"\")"=w346) -> ("States Out"=w345:string)  [unwired: 13 in]
      }
      frame "Send Byte Data" {
        w360 = u32 42  # Bus Idle Timeout
        w367 = u8 225  # ACK
        w374 = u8 227  # ETX
        w377 = u8 226  # STX
        # "Washer ACM Control\t0x25\nWasher MC Control\t0x21\nInverter Control\t0x3F"
        n128 = local read "Byte Data"() -> (w352:u8[])
        n129 = Unbundle By Name(w365) -> ("ComPort"=w357:refnum<visa-resource-name>)
        n130 = local read "Destination Address"() -> (w354:u8)
        n131 = local read "Source Address"() -> (w351:u8)
        n132 = Array Size(array=w352) -> (size(s)=w380:i32)
        n133 = Compound Arithmetic op=ADD(7 ("x"), w380) -> (w378:i32)
        n134 = To Unsigned Byte Integer(number=w378) -> (unsigned 8bit integer=w379:u8)
        n135 = Build Array (concatenate)(w354, w379, w351, w352) -> (w376:u8[])
        n136 = call "crc16-ccitt (x1021).vi"("unsigned byte array"=w376) -> ("CRC"=w375:u8[])  [unwired: 9 in, 1 out]
        n137 = Build Array (concatenate)(w377, w376, w375, w374) -> (w362:u8[])
        n138 = call "GEA2 Add ESC Char.vi"("Message"=w362) -> ("Message Out"=w350:u8[])  [unwired: 14 in]
        n139 = local write "Command Bytes"(w350) -> ()
        n140 = call "GEA2 Wait for Bus Idle.vi"("Error In"=w369, "Idle Time"=w360, "ComPort"=w357) -> ("error out"=w359:errorcluster)  [unwired: 7 in, 1 out]
        n141 = Byte Array To String(unsigned byte array=w350) -> (string=w363:string)
        n142 = Array Size(array=w350) -> (size(s)=w371:i32)
        n143 = VISA Flush I/O Buffer(VISA resource name=w357, error in (no error)=w359) -> (error out=w358:errorcluster)  [unwired: 1 in, 1 out]
        n144 = Increment(x=w371) -> (x+1=w368:i32)
        n145 = VISA Write(VISA resource name=w357, write buffer=w363, error in (no error)=w358) -> (VISA resource name out=w373:refnum<visa-resource-name>, error out=w372:errorcluster)  [unwired: 1 out]
        n146 = To Unsigned Long Integer(number=w368) -> (unsigned 32bit integer=w361:u32)
        n147 = Build Array (concatenate)(w350, w367) -> (w366:u8[])
        n148 = Byte Array To String(unsigned byte array=w366) -> (string=w370:string)
        n149 = VISA Read(VISA resource name=w373, byte count=w361, error in (no error)=w372) -> (read buffer=w356:string, error out=w355:errorcluster)  [unwired: 2 out]
        n150 = case shown="True" "Read?" {
          tunnel: ["" "ReadData\nData: Parse\n"] -> w364
          frame False {
          }
          frame True {
          }
        }
        n151 = Equal?(x=w370, y=w356) -> (x = y?=w349:bool)
        n152 = local write "WriteOK"(w349) -> ()
        n153 = call <vilib>:"Add State(s) to Queue__jki_lib_state_machine.vi"("State(s) in Front (\"\")"=w364, "State(s) in (\"\")"=w383) -> ("States Out"=w382:string)  [unwired: 13 in]
      }
      frame "ReadData" {
        w403 = -1073807252  # Buffer Overflow
        w410 = errorcluster {"status"=TRUE, "code"=-1073807339, "source"="VISA Read in GEA2_ICP_Dryer_SM.vi"}  # timeout error
        # "Try to make sure not in mid of transmission"
        # "Read the port:"
        n154 = Unbundle By Name(w397) -> ("ComPort"=w389:refnum<visa-resource-name>)
        n155 = Unbundle By Name(w397) -> ("Partial Message Start"=w393:u8[])
        n156 = call "GEA2 Wait for Bus Idle.vi"("Error In"=w391, "Idle Time"="Read Bus Idle Timeout", "ComPort"=w389) -> ("error out"=w392:errorcluster, "Bytes at Port"=w390:u32)  [unwired: 7 in]
        n157 = Array Size(array=w393) -> (size(s)=w396:i32)
        n158 = To Unsigned Long Integer(number=w390) -> (unsigned 32bit integer=w388:u32)
        "Bytes At Port" <- w388
        n159 = To Long Integer(number=w388) -> (32bit integer=w386:i32)
        n160 = Add(x=w396, y=w386) -> (x+y=w395:i32)
        n161 = VISA Read(VISA resource name=w389, byte count=w388, error in (no error)=w392) -> (read buffer=w412:string, error out=w404:errorcluster)  [unwired: 2 out]
        n162 = Unbundle By Name(w404) -> ("code"=w402:i32)
        n163 = String To Byte Array(string=w412) -> (unsigned byte array=w411:u8[])
        n164 = Build Array (concatenate)(w393, w411) -> (w394:u8[])
        "ReadArray" <- w394
        n165 = Equal?(x=w404, y=w410) -> (x = y?=w409:bool)
        "Timeout" <- w409
        n166 = Equal?(x=w402, y=w403) -> (x = y?=w405:bool)
        n167 = Or(x=w409, y=w405) -> (x .or. y?=w406:bool)
        n168 = case shown="False" w406 {
          tunnel: [w417 w418] -> w400
          tunnel: errorcluster {"status"=FALSE, "code"=0, "source"=""} ("Error Out") -> [_ w418]
          tunnel: w404 -> [w417 _]
          frame False {
          }
          frame True {
          }
        }
        n169 = Bundle By Name(cluster=w397, "Total Bytes Read"=w395, "ReadArray"=w394, "CRCArray"=u8[] [] ("ReadArray"), "Current Read Index"=0) -> (w407:T7)
        n170 = local read "Exit"() -> (w399:bool)
        n171 = case shown="True" w399 {
          tunnel: [_ "Exit" ("State(s) in Front (\"\")")] -> w398
          frame False {
          }
          frame True {
          }
        }
        n172 = call <vilib>:"Add State(s) to Queue__jki_lib_state_machine.vi"("State(s) in Front (\"\")"=w398, "State(s) in (\"\")"=w415) -> ("States Out"=w414:string)  [unwired: 13 in]
      }
      frame " ------- ReadData ------------ " {
        # "Template Separator\n(You can make a copy of, or modify, this frame)"
        n173 = call <vilib>:"Add State(s) to Queue__jki_lib_state_machine.vi"("State(s) in (\"\")"=w422) -> ("States Out"=w421:string)  [unwired: 14 in]
      }
      frame "Data: Parse" {
        # "Template Separator\n(You can make a copy of, or modify, this frame)"
        n174 = Unbundle By Name(w425) -> ("Total Bytes Read"=w423:i32)
        n175 = To Long Integer(number=w423) -> (32bit integer=w427:i32)
        n176 = Equal To 0?(x=w427) -> (x = 0?=w426:bool)
        n177 = case shown="False" w426 {
          tunnel: ["Interpret Bytes" ("State(s) in Front (\"\")") "Parse: STX\nParse: Destination\nParse: Length\nParse: Source\nParse: Bytes Data\nParse: CRC1\nParse: CRC2\nCheckCRC\nParse: ETX\nInterpret Bytes\nCheck Complete" ("State(s) in Front (\"\")")] -> w428
          tunnel: w425 -> [w434 w436]
          tunnel: [w433 w436] -> w424
          frame True {
            n178 = Bundle By Name(cluster=w434, "Bytes Data"=u8[] []) -> (w433:T7)
          }
          frame False {
          }
        }
        n179 = call <vilib>:"Add State(s) to Queue__jki_lib_state_machine.vi"("State(s) in Front (\"\")"=w428, "State(s) in (\"\")"=w431) -> ("States Out"=w430:string)  [unwired: 13 in]
      }
      frame "Parse: STX" {
        # "Your code here.\n(You can make a copy of, or modify, this frame)"
        n180 = Unbundle By Name(w450) -> ("Total Bytes Read"=w442:i32, "Current Read Index"=w443:i32, "ReadArray"=w438:u8[])
        n181 = while {
          tunnel: [w459] -> w448
          tunnel: w442 -> [w458]
          shift-right: [w456] -> w441
          shift-left: w443 -> [w453]
          tunnel: w438 -> [w461]
          tunnel: [w453] -> w440
          stop <- w460 stop-if-true
          w455 = u8 226  # STX
          n182 = Increment(x=w453) -> (x+1=w456:i32)
          n183 = Index Array(array=w461, index=w453) -> (element=w454:u8)
          n184 = Less?(x=w458, y=w456) -> (x < y?=w457:bool)
          n185 = Equal?(x=w454, y=w455) -> (x = y?=w459:bool)
          n186 = Or(x=w457, y=w459) -> (x .or. y?=w460:bool)
        }
        n187 = case shown="False" w448 {
          tunnel: w445 -> [w467 w469]
          tunnel: [w465 w469] -> w447
          tunnel: ["Exit" ("State(s) in Front (\"\")") _] -> w446
          tunnel: w440 -> [_ w468]
          tunnel: [0 ("Current Start of Message Index") w468] -> w439
          frame False {
            n188 = Bundle By Name(cluster=w467, "source"="Partial GEA Message") -> (w465:errorcluster)
            n189 = local write "Partial Message"(TRUE ("Partial Message")) -> ()
          }
          frame True {
          }
        }
        "Current Start of Message Index" <- w439
        n190 = Bundle By Name(cluster=w450, "Current Read Index"=w441, "Bytes Data"=u8[] []) -> (w449:T7)
        n191 = call <vilib>:"Add State(s) to Queue__jki_lib_state_machine.vi"("State(s) in Front (\"\")"=w446, "State(s) in (\"\")"=w452) -> ("States Out"=w451:string)  [unwired: 13 in]
      }
      frame "Parse: Source" {
        w480 = u8 224  # ESC
        n192 = Unbundle By Name(w482) -> ("CRCArray"=w477:u8[], "ReadArray"=w473:u8[], "Current Read Index"=w475:i32)  [unwired: 1 out]
        n193 = Increment(x=w475) -> (x+1=w472:i32)
        n194 = Index Array(array=w473, index=w475) -> (element=w474:u8)
        n195 = Equal?(x=w474, y=w480) -> (x = y?=w479:bool)
        n196 = case shown="True" w479 {
          tunnel: [w486 w489] -> w470
          tunnel: [w485 w487] -> w471
          tunnel: w473 -> [_ w490]
          tunnel: w474 -> [w486 _]
          tunnel: w472 -> [w485 w488]
          frame False {
          }
          frame True {
            n197 = Increment(x=w488) -> (x+1=w487:i32)
            n198 = Index Array(array=w490, index=w488) -> (element=w489:u8)
          }
        }
        "Source Read" <- w470
        n199 = Build Array (concatenate)(w477, w470) -> (w476:u8[])
        n200 = Bundle By Name(cluster=w482, "CRCArray"=w476, "Current Read Index"=w471) -> (w481:T7)
        n201 = call <vilib>:"Add State(s) to Queue__jki_lib_state_machine.vi"("State(s) in (\"\")"=w484) -> ("States Out"=w483:string)  [unwired: 14 in]
      }
      frame "Parse: Length" {
        w513 = -3  # CRC + ETX
        w501 = u8 224  # ESC
        n202 = Unbundle By Name(w519) -> ("Total Bytes Read"=w508:i32, "ReadArray"=w494:u8[], "CRCArray"=w514:u8[], "Current Read Index"=w493:i32)  [unwired: 1 out]
        n203 = Increment(x=w493) -> (x+1=w510:i32)
        n204 = Index Array(array=w494, index=w493) -> (element=w509:u8)
        n205 = Equal?(x=w509, y=w501) -> (x = y?=w517:bool)
        n206 = case shown="True" w517 {
          tunnel: [w526 w528] -> w492
          tunnel: [w527 w529] -> w506
          tunnel: w494 -> [_ _]
          tunnel: w494 -> [_ w531]
          tunnel: w510 -> [w527 w530]
          tunnel: w509 -> [w526 _]
          frame False {
          }
          frame True {
            n207 = Index Array(array=w531, index=w530) -> (element=w528:u8)
            n208 = Increment(x=w530) -> (x+1=w529:i32)
          }
        }
        "Length" <- w492
        n209 = Array Subset(array=w494, index=w493, length=w492) -> (w491:u8[])
        n210 = Equal?(x=w491, y=w501) -> (x = y?=w500:bool[])
        n211 = Boolean To (0,1)(Boolean=w500) -> (0, 1=w499:i16[])
        n212 = Add Array Elements(numeric array=w499) -> (sum=w498:i16)
        n213 = Multiply(x=w498, y=i16 -1) -> (x*y=w496:i16)
        n214 = To Long Integer(number=w496) -> (32bit integer=w495:i32)
        n215 = Build Array (concatenate)(w514, w492) -> (w515:u8[])
        n216 = Bundle By Name(cluster=w519, "Current Read Index"=w506, "CRCArray"=w515, "Bytes Remaining"=w492) -> (w518:T7)
        n217 = To Long Integer(number=w492) -> (32bit integer=w505:i32)
        n218 = Compound Arithmetic op=ADD(w506, w513, w505, w495) -> (w512:i32)
        n219 = To Long Integer(number=w512) -> (32bit integer=w507:i32)
        n220 = Less?(x=w508, y=w507) -> (x < y?=w511:bool)
        "Partial Message" <- w511
        n221 = local read "Mode"() -> (w504:T2)
        n222 = case shown="True" w511 {
          tunnel: w504 -> [_ w523]
          tunnel: [w521 w522] -> w502
          tunnel: w503 -> [w521 _]
          frame False {
          }
          frame True {
            n223 = case shown="\"Init Com Port\", Default" w523 {
              tunnel: ["Partial Message\nExit" ("State(s) in Front (\"\")") "Read Continue" ("State(s) in Front (\"\")")] -> w522
              frame "Init Com Port", Default {
              }
              frame "Read Continuous" {
              }
            }
          }
        }
        n224 = call <vilib>:"Add State(s) to Queue__jki_lib_state_machine.vi"("State(s) in (\"\")"=w502) -> ("States Out"=w520:string)  [unwired: 14 in]
      }
      frame "Parse: Destination" {
        w541 = u8 224  # ESC
        n225 = Unbundle By Name(w545) -> ("ReadArray"=w532:u8[], "Current Read Index"=w537:i32)
        n226 = Increment(x=w537) -> (x+1=w536:i32)
        n227 = Index Array(array=w532, index=w537) -> (element=w533:u8)
        n228 = Equal?(x=w533, y=w541) -> (x = y?=w540:bool)
        n229 = case shown="True" w540 {
          tunnel: [w549 w550] -> w535
          tunnel: [w548 w552] -> w538
          tunnel: w532 -> [_ w553]
          tunnel: w536 -> [w548 w551]
          tunnel: w533 -> [w549 _]
          frame False {
          }
          frame True {
            n230 = Index Array(array=w553, index=w551) -> (element=w550:u8)
            n231 = Increment(x=w551) -> (x+1=w552:i32)
          }
        }
        "Destination Read" <- w535
        n232 = local read "Source Address"() -> (w542:u8)
        n233 = Build Array(w535) -> (w534:u8[])
        n234 = Bundle By Name(cluster=w545, "Current Read Index"=w538, "CRCArray"=w534) -> (w544:T7)
        n235 = Equal?(x=w535, y=w542) -> (x = y?=→"Message for Me":bool)
        n236 = call <vilib>:"Add State(s) to Queue__jki_lib_state_machine.vi"("State(s) in (\"\")"=w547) -> ("States Out"=w546:string)  [unwired: 14 in]
      }
      frame "Parse: Bytes Data" {
        w572 = u8 224  # ESC
        n237 = Unbundle By Name(w574) -> ("ReadArray"=w557:u8[], "CRCArray"=w568:u8[], "Bytes Remaining"=w567:u8, "Bytes Data"=w565:u8[], "Current Read Index"=w556:i32)
        n238 = Increment(x=w556) -> (x+1=w555:i32)
        n239 = Index Array(array=w557, index=w556) -> (element=w554:u8)
        n240 = Equal?(x=w554, y=w572) -> (x = y?=w571:bool)
        n241 = case shown="True" w571 {
          tunnel: [w578 w580] -> w563
          tunnel: [w579 w583] -> w566
          tunnel: w557 -> [_ w582]
          tunnel: w557 -> [_ _]
          tunnel: w555 -> [w579 w581]
          tunnel: w554 -> [w578 _]
          frame False {
          }
          frame True {
            n242 = Index Array(array=w582, index=w581) -> (element=w580:u8)
            n243 = Increment(x=w581) -> (x+1=w583:i32)
          }
        }
        n244 = Decrement(x=w567) -> (x-1=w560:u8)
        n245 = Build Array (concatenate)(w565, w563) -> (w564:u8[])
        n246 = Build Array (concatenate)(w568, w563) -> (w569:u8[])
        n247 = Subtract(x=w560, y=u8 7) -> (x-y=w558:u8)
        n248 = Bundle By Name(cluster=w574, "Current Read Index"=w566, "CRCArray"=w569, "Bytes Remaining"=w560, "Bytes Data"=w564) -> (w573:T7)
        n249 = Greater Than 0?(x=w558) -> (x > 0?=w562:bool)
        n250 = case shown="True" w562 {
          tunnel: [_ "Parse: Bytes Data" ("State(s) in Front (\"\")")] -> w561
          frame False {
          }
          frame True {
          }
        }
        n251 = call <vilib>:"Add State(s) to Queue__jki_lib_state_machine.vi"("State(s) in Front (\"\")"=w561, "State(s) in (\"\")"=w576) -> ("States Out"=w575:string)  [unwired: 13 in]
      }
      frame "Parse: CRC1" {
        w593 = u8 224  # ESC
        n252 = Unbundle By Name(w595) -> ("ReadArray"=w588:u8[], "Current Read Index"=w587:i32)  [unwired: 1 out]
        n253 = Increment(x=w587) -> (x+1=w586:i32)
        n254 = Index Array(array=w588, index=w587) -> (element=w585:u8)
        n255 = Equal?(x=w585, y=w593) -> (x = y?=w592:bool)
        n256 = case shown="True" w592 {
          tunnel: [w598 w600] -> w589
          tunnel: [w599 w603] -> w590
          tunnel: w588 -> [_ w602]
          tunnel: w586 -> [w599 w601]
          tunnel: w585 -> [w598 _]
          frame False {
          }
          frame True {
            n257 = Index Array(array=w602, index=w601) -> (element=w600:u8)
            n258 = Increment(x=w601) -> (x+1=w603:i32)
          }
        }
        n259 = Build Array(w589) -> (w584:u8[])
        n260 = Bundle By Name(cluster=w595, "Current Read Index"=w590, "CRCRead"=w584) -> (w594:T7)
        n261 = call <vilib>:"Add State(s) to Queue__jki_lib_state_machine.vi"("State(s) in (\"\")"=w597) -> ("States Out"=w596:string)  [unwired: 14 in]
      }
      frame "Parse: CRC2" {
        w614 = u8 224  # ESC
        n262 = Unbundle By Name(w616) -> ("ReadArray"=w605:u8[], "CRCRead"=w608:u8[], "Current Read Index"=w607:i32)
        n263 = Increment(x=w607) -> (x+1=w606:i32)
        n264 = Index Array(array=w605, index=w607) -> (element=w604:u8)
        n265 = Equal?(x=w604, y=w614) -> (x = y?=w613:bool)
        n266 = case shown="True" w613 {
          tunnel: [w619 w621] -> w610
          tunnel: [w620 w624] -> w611
          tunnel: w605 -> [_ w623]
          tunnel: w606 -> [w620 w622]
          tunnel: w604 -> [w619 _]
          frame False {
          }
          frame True {
            n267 = Increment(x=w622) -> (x+1=w624:i32)
            n268 = Index Array(array=w623, index=w622) -> (element=w621:u8)
          }
        }
        n269 = Build Array (concatenate)(w608, w610) -> (w609:u8[])
        n270 = Bundle By Name(cluster=w616, "Current Read Index"=w611, "CRCRead"=w609) -> (w615:T7)
        n271 = call <vilib>:"Add State(s) to Queue__jki_lib_state_machine.vi"("State(s) in (\"\")"=w618) -> ("States Out"=w617:string)  [unwired: 14 in]
      }
      frame "CheckCRC" {
        # "Your code here.\n(You can make a copy of, or modify, this frame)"
        n272 = Unbundle By Name(w629) -> ("CRCRead"=w626:u8[], "CRCArray"=w631:u8[])  [unwired: 2 out]
        "CRCRead" <- w626
        "CRCArray" <- w631
        n273 = call "crc16-ccitt (x1021).vi"("error in (no error)"=w632, "unsigned byte array"=w631) -> ("error out (dup)"=w627:errorcluster, "CRC"=w630:u8[])  [unwired: 8 in]
        "CRC Calc" <- w630
        n274 = Equal?(x=w626, y=w630) -> (x = y?=w625:bool)
        "CRC Match" <- w625
        n275 = Bundle By Name(cluster=w629, "CRC"=w625) -> (w628:T7)
        n276 = call <vilib>:"Add State(s) to Queue__jki_lib_state_machine.vi"("State(s) in (\"\")"=w634) -> ("States Out"=w633:string)  [unwired: 14 in]
      }
      frame "Parse: ETX" {
        w635 = u8 227  # ETX
        # "Your code here.\n(You can make a copy of, or modify, this frame)"
        n277 = Unbundle By Name(w645) -> ("ReadArray"=w640:u8[], "Current Read Index"=w636:i32)
        n278 = Index Array(array=w640, index=w636) -> (element=w638:u8)
        n279 = Increment(x=w636) -> (x+1=w637:i32)
        n280 = Equal?(x=w638, y=w635) -> (x = y?=w643:bool)
        n281 = case shown="False" w643 {
          tunnel: w639 -> [w651 w653]
          tunnel: [w648 w653] -> w642
          tunnel: ["Exit" ("State(s) in Front (\"\")") _] -> w641
          frame False {
            n282 = call "Error Bool Enumerator.vi"("Error Enum"=HEWH_Error_Enumeration."GEA2 ETX", "Error In"=w651, "Error?"=TRUE) -> ("Error Out"=w648:errorcluster)  [unwired: 6 in]
          }
          frame True {
          }
        }
        n283 = Bundle By Name(cluster=w645, "Current Read Index"=w637) -> (w644:T7)
        n284 = call <vilib>:"Add State(s) to Queue__jki_lib_state_machine.vi"("State(s) in Front (\"\")"=w641, "State(s) in (\"\")"=w647) -> ("States Out"=w646:string)  [unwired: 13 in]
      }
      frame "SendACK" {
        # "Not called, since reading all at once..."
        n285 = Unbundle By Name(w655) -> ("ComPort"=w657:refnum<visa-resource-name>, "CRC"=w654:bool)
        n286 = case shown="True" w654 {
          tunnel: w658 -> [w661 w663]
          tunnel: w657 -> [_ w662]
          tunnel: [w661 w667] -> w656
          frame False {
          }
          frame True {
            n287 = local read "Destination Read"() -> (w666:u8)
            n288 = local read "Source Address"() -> (w665:u8)
            n289 = Equal?(x=w665, y=w666) -> (x = y?=w664:bool)
            n290 = case shown="True" w664 {
              tunnel: w663 -> [w668 w673]
              tunnel: [w668 w676] -> w667
              tunnel: w662 -> [_ w670]
              frame False {
                # "Skip Readback"
              }
              frame True {
                w675 = u8 225  # ACK
                n291 = Build Array(w675) -> (w674:u8[])
                n292 = Byte Array To String(unsigned byte array=w674) -> (string=w669:string)
                n293 = VISA Write(VISA resource name=w670, write buffer=w669, error in (no error)=w673) -> (VISA resource name out=w671:refnum<visa-resource-name>, error out=w672:errorcluster)  [unwired: 1 out]
                n294 = VISA Read(VISA resource name=w671, byte count=u32 1, error in (no error)=w672) -> (read buffer=w678:string, error out=w676:errorcluster)  [unwired: 2 out]
                n295 = Equal?(x=w669, y=w678) -> (x = y?=→"Read_ACK":bool)
              }
            }
          }
        }
        n296 = call <vilib>:"Add State(s) to Queue__jki_lib_state_machine.vi"("State(s) in (\"\")"=w660) -> ("States Out"=w659:string)  [unwired: 14 in]
      }
      frame "Interpret Bytes" {
        # "Template Separator\n(You can make a copy of, or modify, this frame)"
        n297 = Unbundle By Name(w683) -> ("Bytes Data"=w688:u8[], "CRC"=w686:bool, "Good Responses"=w684:cluster{"Bytes Data":u8[]}[])
        "DataReturned" <- w688
        n298 = case shown="False" "Filter on Destination" {
          tunnel: [TRUE ("Message for Me") w693] -> w687
          frame False {
          }
          frame True {
            n299 = local read "Message for Me"() -> (w693:bool)
          }
        }
        n300 = And(x=w686, y=w687) -> (x .and. y?=w685:bool)
        n301 = case shown="True" w685 {
          tunnel: w688 -> [_ w698]
          tunnel: [w694 w696] -> w681
          tunnel: w684 -> [w694 w695]
          frame False {
          }
          frame True {
            n302 = Bundle By Name(cluster=cluster{"Bytes Data":u8[]} {"Bytes Data"=[]} ("Cluster"), "Bytes Data"=w698) -> (w697:cluster{"Bytes Data":u8[]})
            n303 = Build Array (concatenate)(w695, w697) -> (w696:cluster{"Bytes Data":u8[]}[])
          }
        }
        "Good Responses" <- w681
        n304 = Bundle By Name(cluster=w683, "Good Responses"=w681) -> (w682:T7)
        n305 = call <vilib>:"Add State(s) to Queue__jki_lib_state_machine.vi"("State(s) in (\"\")"=w691) -> ("States Out"=w690:string)  [unwired: 14 in]
      }
      frame "Check Complete" {
        # "Template Separator\n(You can make a copy of, or modify, this frame)"
        n306 = Unbundle By Name(w702) -> ("Total Bytes Read"=w706:i32, "Current Read Index"=w705:i32, "Reset MSG Count"=w703:bool)
        n307 = Subtract(x=w706, y=w705) -> (x-y=w704:i32)
        n308 = call "Counter.vi"("Reset"=w703) -> ("Count"=→"Num Messages":dbl)  [unwired: 10 in]
        n309 = Greater?(x=w704, y=7) -> (0:w709:bool)
        n310 = case shown="True" w709 {
          tunnel: [_ "Parse: STX\nParse: Destination\nParse: Length\nParse: Source\nParse: Bytes Data\nParse: CRC1\nParse: CRC2\nCheckCRC\nParse: ETX\nInterpret Bytes\nCheck Complete" ("State(s) in Front (\"\")")] -> w708
          frame False {
          }
          frame True {
          }
        }
        n311 = Bundle By Name(cluster=w702, "Reset MSG Count"=FALSE) -> (w701:T7)
        n312 = call <vilib>:"Add State(s) to Queue__jki_lib_state_machine.vi"("State(s) in Front (\"\")"=w708, "State(s) in (\"\")"=w713) -> ("States Out"=w712:string)  [unwired: 13 in]
      }
      frame "Read Continue" {
        # "Template Separator\n(You can make a copy of, or modify, this frame)"
        n313 = Unbundle By Name(w721) -> ("Reset Pulse"=w720:bool)
        n314 = call "Counter.vi"("Reset"=w720) -> ("Count"=→"Read Message Count":dbl)  [unwired: 10 in]
        n315 = local read "Read Continuous"() -> (w715:bool)
        n316 = case shown="False" w715 {
          tunnel: [_ "ReadData\nData: Parse\nRead Continue"] -> w718
          frame False {
          }
          frame True {
          }
        }
        n317 = Bundle By Name(cluster=w721, "Reset Pulse"=FALSE ("Reset MSG Count")) -> (w724:T7)
        n318 = local read "Exit"() -> (w719:bool)
        n319 = Select(t="Exit", s=w719, f=w718) -> (s? t:f=w716:string)
        n320 = call <vilib>:"Add State(s) to Queue__jki_lib_state_machine.vi"("State(s) in Front (\"\")"=w716, "State(s) in (\"\")"=w727) -> ("States Out"=w726:string)  [unwired: 13 in]
      }
      frame "Partial Message" {
        n321 = Unbundle By Name(w732) -> ("ReadArray"=w731:u8[])
        n322 = local read "Current Start of Message Index"() -> (w730:i32)
        n323 = Array Subset(array=w731, index=w730) -> (→"Partial Message Out":u8[])  [unwired: 1 in]
        n324 = call <vilib>:"Add State(s) to Queue__jki_lib_state_machine.vi"("State(s) in (\"\")"=w734) -> ("States Out"=w735:string)  [unwired: 14 in]
      }
    }
    n325 = Equal To 0?(x=w34) -> (x = 0?=w33:bool)
    n326 = case shown="False" "Debug" {
      tunnel: w37 -> [_ w52]
      tunnel: w33 -> [_ w51]
      frame False {
      }
      frame True {
        n327 = call "Build String Array w Max Size.vi"("Initialize"=w51, "string"=w52) -> ("Array"=→"State Array":string[])  [unwired: 9 in]
      }
    }
    n328 = local write "Error Out"(w42) -> ()
    n329 = flat-sequence {
      tunnel: [w55] -> w41
      tunnel: w42 -> [_]
      tunnel: [w54] -> w40
      frame #0 {
        n330 = local read "tStart"() -> (w54:u32)
        n331 = Tick Count (ms)() -> (millisecond timer value=w55:u32)
      }
    }
    n332 = To Long Integer(number=w41) -> (32bit integer=w39:i32)
    n333 = To Long Integer(number=w40) -> (32bit integer=w38:i32)
  }
  n334 = local read "Debug"() -> (w3:bool)
  n335 = case shown="True" w3 {
    tunnel: w9 -> [_ w739]
    tunnel: w8 -> [_ w738]
    frame False {
    }
    frame True {
      n336 = Subtract(x=w739, y=w738) -> (x-y=w740:i32[])
      "Time Array" <- w740
      n337 = Delete From Array(array=w740, length=1, index=0) -> (array with subset deleted=w741:i32[])  [unwired: 1 out]
      n338 = for {
        tunnel: w741 -> [w746] mode=indexing
        tunnel: w740 -> [w745] mode=indexing
        tunnel: [w744] -> w737 mode=indexing
        n339 = Subtract(x=w746, y=w745) -> (x-y=w744:i32)
      }
      "Tdiff" <- w737
      n340 = Add Array Elements(numeric array=w737) -> (sum=→"Total mS":i32)
    }
  }
  n341 = Unbundle By Name(w6) -> ("Error Out Flag"=w5:bool)
  n342 = Bundle By Name(cluster=w10, "status"=w5) -> (→"Error Out":errorcluster)
